vi "mapV2.vi"() -> ()   [LabVIEW 2024]
uses:
  D:/Autonomous Systems/Oulu/Measurment Systems/Examples/GMap.NET/GMapControl/GMapControl/bin/Debug/GMapControl.dll
  GMap.NET/GMapControl/GMapControl/bin/Debug/GMapControl.dll
panel:
  out "GetLatitude":dbl
  in  "MapControl":refnum<k24>(container)
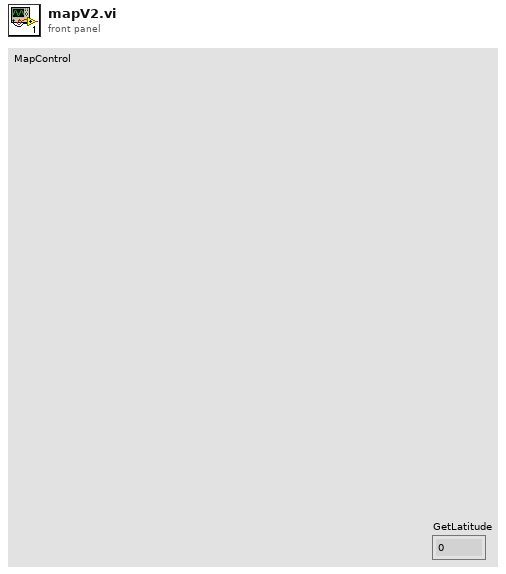
[diagram p1: front panel]
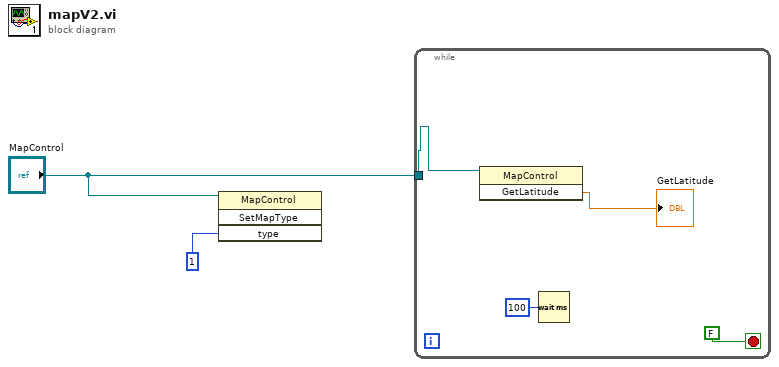
[diagram p0: block diagram]
diagram:
  n1 = invoke class="MapControl" method="SetMapType"(reference="MapControl", "type"=1) -> ()  [unwired: 2 in, 4 out]
  n2 = while {
    tunnel: "MapControl" -> [w4]
    stop <- FALSE stop-if-true
    n3 = invoke class="MapControl" method="GetLatitude"(reference=w4) -> ("GetLatitude"=→"GetLatitude":dbl)  [unwired: 2 in, 2 out]
    n4 = Wait (ms)(milliseconds to wait=u32 100) -> ()  [unwired: 1 out]
  }
